vi "ByteTransfer.vi"(8 "error in":errorcluster, 9 "Packet Size":u32, 11 "VISA resource name":refnum<visa-resource-name>="COM1") -> (0 "error out":errorcluster, 3 "Command Echo":u8[](array[numeric]))   [LabVIEW 2019]
panel:
  out "read buffer":string
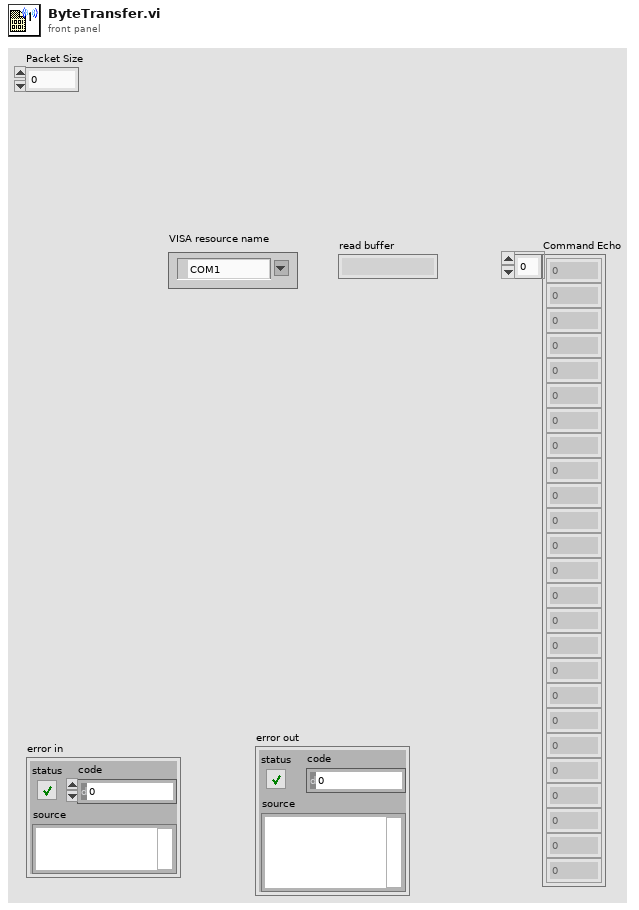
[diagram p1: front panel]
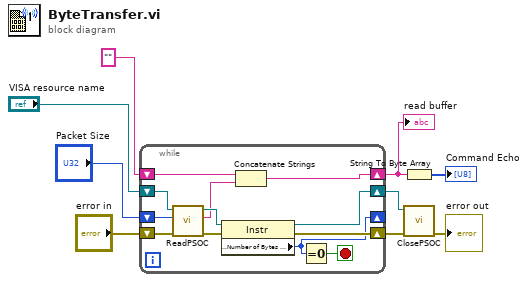
[diagram p0: block diagram]
diagram:
  n1 = while {
    shift-right: [w17] -> w6
    shift-left: "VISA resource name" -> [w21]
    shift-right: [w15] -> w9
    shift-left: "error in" -> [w19]
    shift-right: [w12] -> w5
    shift-left: "" -> [w11]
    shift-right: [w10] -> _
    shift-left: "Packet Size" -> [w20]
    stop <- w14 stop-if-true
    n2 = call "ReadPSOC.vi"("error in"=w19, "byte count"=w20, "VISA resource name"=w21) -> ("error out"=w16:errorcluster, "read buffer"=w13:string, "VISA resource name out"=w18:refnum<visa-resource-name>)  [unwired: 5 in]
    n3 = property class="Instr"(reference=w18, error in=w16) -> (reference out=w17:refnum<visa-resource-name>, error out=w15:errorcluster, "Serial Settings:Number of Bytes at Serial Port"=w10:u32)
    n4 = Concatenate Strings(w11, w13) -> (w12:string)
    n5 = Equal To 0?(x=w10) -> (x = 0?=w14:bool)
  }
  "read buffer" <- w5
  n6 = String To Byte Array(string=w5) -> (unsigned byte array=→"Command Echo":u8[])
  n7 = call "ClosePSOC.vi"("error in"=w9, "VISA resource name"=w6) -> ("error out"=→"error out":errorcluster)  [unwired: 9 in]
